vi "Indexing_Modbus.vi"(0 "Modbus master in":refnum<class "Modbus Master.lvclass">, 1 "Index Parameters":cluster{"Index":bool, "Start Index":bool}, 2 "Index Timeout":u16, 3 "Index Position":u16[](array[numeric]), 4 "Index Hardware Torque Limit":u16, 5 "Index Software Torque Limit":u16, 7 "error in (no error)":errorcluster) -> (20 "Modbus master out":refnum<class "Modbus Master.lvclass">, 27 "error out":errorcluster)   [LabVIEW 2021]
uses:
  <vilib>/Modbus/master/Modbus Master.lvclass
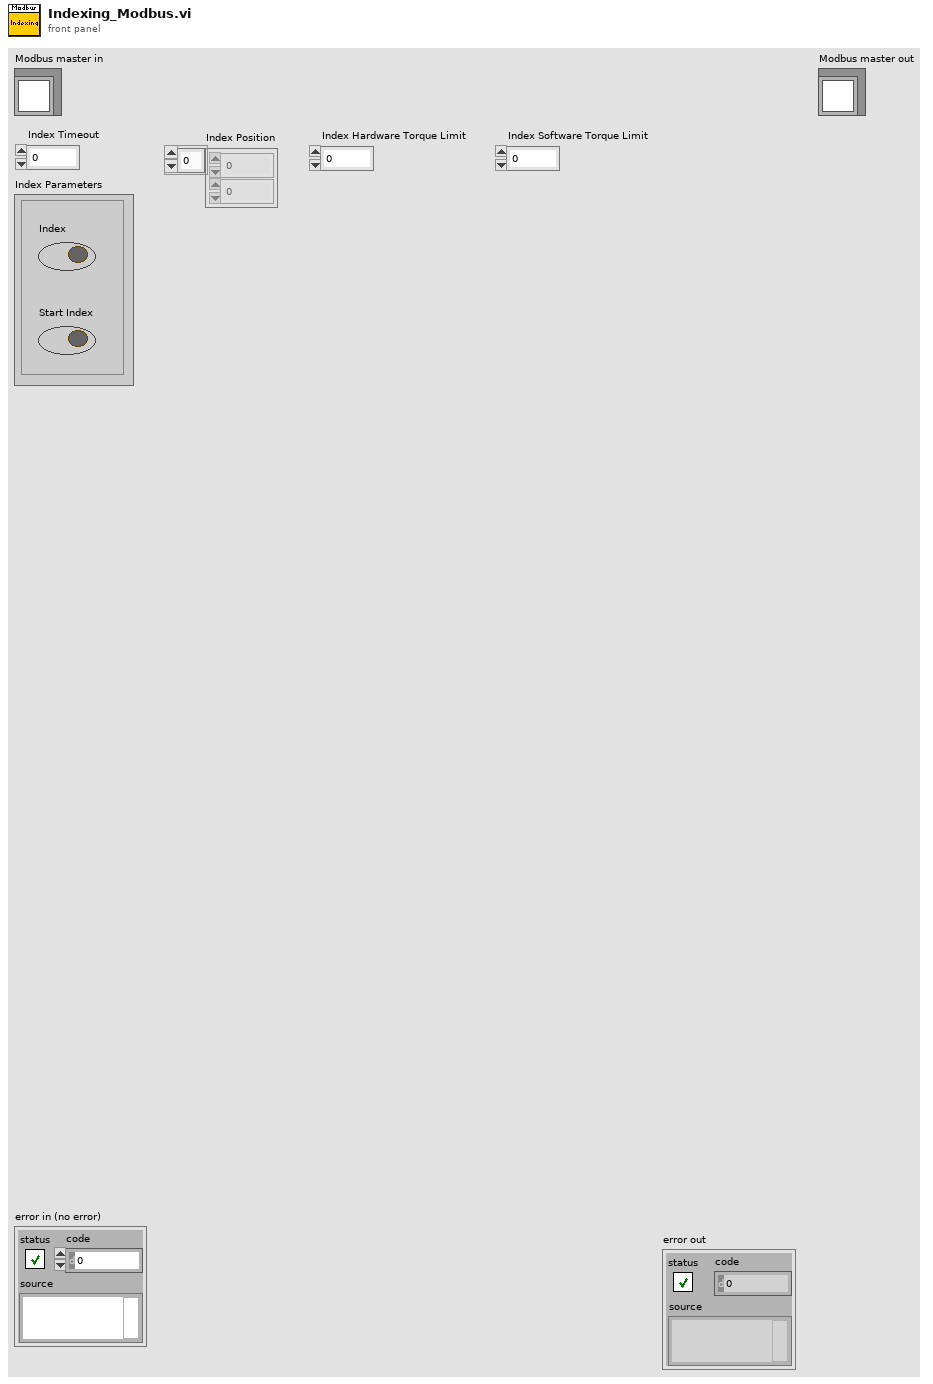
[diagram p1: front panel]
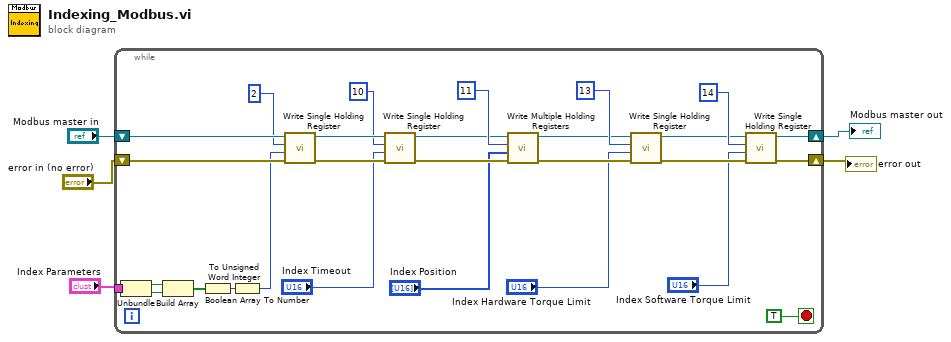
[diagram p0: block diagram]
diagram:
  n1 = while {
    tunnel: "Index Parameters" -> [w30]
    shift-right: [w8] -> w2
    shift-left: "Modbus master in" -> [w33]
    shift-right: [w7] -> w1
    shift-left: "error in (no error)" -> [w32]
    stop <- TRUE stop-if-true
    n2 = Unbundle(w30) -> ("Index"=w28:bool, "Start Index"=w29:bool)
    n3 = Build Array(w28, w29) -> (w27:bool[])
    n4 = Boolean Array To Number(Boolean array=w27) -> (number=w26:u32)
    n5 = To Unsigned Word Integer(number=w26) -> (unsigned 16bit integer=w25:u16)
    n6 = call-dynamic "Write Single Holding Register.vi"("error in (no error)"=w32, "holding register value"=w25, "address"=u16 2, "Modbus master in"=w33) -> ("error out"=w23:errorcluster, "Modbus master out"=w24:refnum<class "Modbus Master.lvclass">)  [unwired: 6 in]
    n7 = call-dynamic "Write Single Holding Register.vi"("error in (no error)"=w23, "holding register value"="Index Timeout", "address"=u16 10, "Modbus master in"=w24) -> ("error out"=w18:errorcluster, "Modbus master out"=w19:refnum<class "Modbus Master.lvclass">)  [unwired: 6 in]
    n8 = call-dynamic "Write Multiple Holding Registers.vi"("error in (no error)"=w18, "holding register values"="Index Position", "starting address"=u16 11, "Modbus master in"=w19) -> ("error out"=w14:errorcluster, "Modbus master out"=w13:refnum<class "Modbus Master.lvclass">)  [unwired: 6 in]
    n9 = call-dynamic "Write Single Holding Register.vi"("error in (no error)"=w14, "holding register value"="Index Hardware Torque Limit", "address"=u16 13, "Modbus master in"=w13) -> ("error out"=w11:errorcluster, "Modbus master out"=w12:refnum<class "Modbus Master.lvclass">)  [unwired: 6 in]
    n10 = call-dynamic "Write Single Holding Register.vi"("error in (no error)"=w11, "holding register value"="Index Software Torque Limit", "address"=u16 14, "Modbus master in"=w12) -> ("error out"=w7:errorcluster, "Modbus master out"=w8:refnum<class "Modbus Master.lvclass">)  [unwired: 6 in]
  }
  "Modbus master out" <- w2
  "error out" <- w1
